vi "Dispose.vi"(8 "error in (no error)":errorcluster, 11 "TwinCAT ADS in":refnum<class "TwinCAT ADS.lvclass">) -> (0 "error out":errorcluster)   [LabVIEW 2018, in "TwinCAT ADS.lvclass"]
uses:
  TwinCAT ADS.lvclass
  TwinCAT ADS.lvclass/TwinCAT ADS.ctl
  TwinCAT.Ads
  Get Type Map.vi
  From Notification Key.vi
  Get Notification Map.vi
  Extensions/Delete Notification By Handle.vi
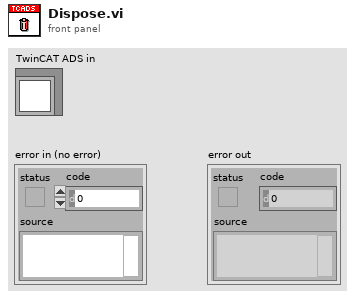
[diagram p1: front panel]
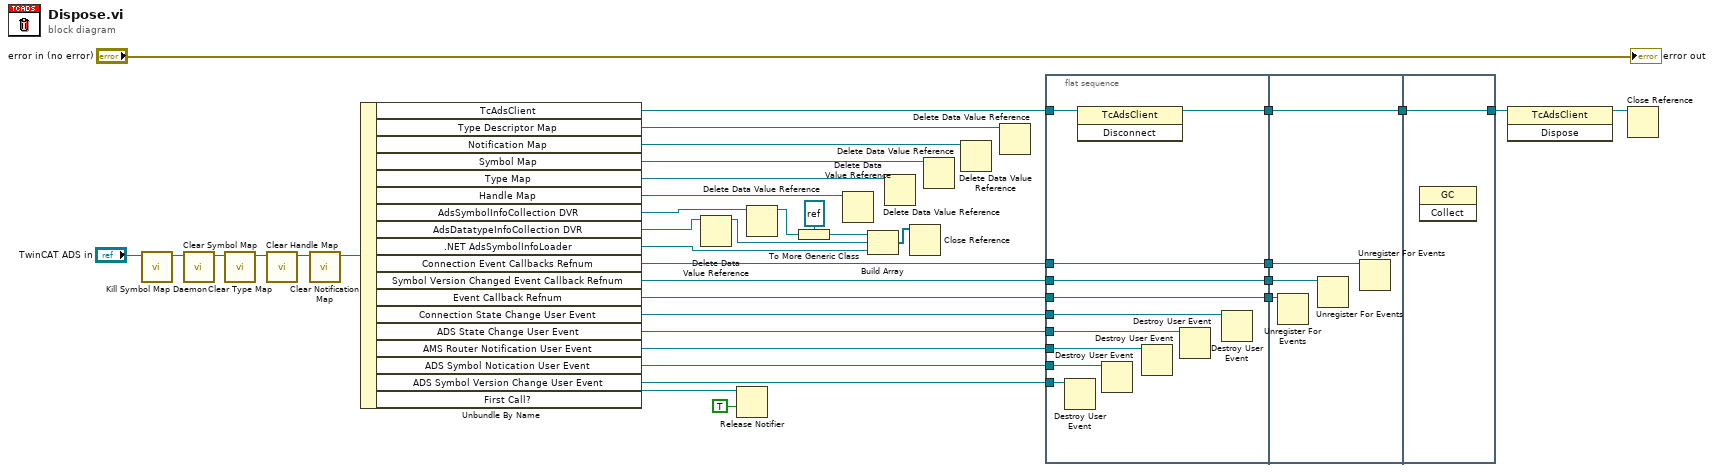
[diagram p0: block diagram]
diagram:
  n1 = call "Kill Symbol Map Daemon.vi"("TwinCAT ADS in"="TwinCAT ADS in") -> ("TwinCAT ADS out"=w3:refnum<class "TwinCAT ADS.lvclass">)  [unwired: 9 in, 1 out]
  n2 = call "Clear Symbol Map.vi"("TwinCAT ADS in"=w3) -> ("TwinCAT ADS out"=w35:refnum<class "TwinCAT ADS.lvclass">)  [unwired: 9 in, 1 out]
  n3 = call "Clear Type Map.vi"("TwinCAT ADS in"=w35) -> ("TwinCAT ADS out"=w34:refnum<class "TwinCAT ADS.lvclass">)  [unwired: 8 in, 2 out]
  n4 = call "Clear Handle Map.vi"("TwinCAT ADS in"=w34) -> ("TwinCAT ADS out"=w7:refnum<class "TwinCAT ADS.lvclass">)  [unwired: 9 in, 1 out]
  n5 = call "Clear Notification Map.vi"("TwinCAT ADS in"=w7) -> ("TwinCAT ADS out"=w6:refnum<class "TwinCAT ADS.lvclass">)  [unwired: 6 in, 4 out]
  n6 = Unbundle By Name(w6) -> ("TcAdsClient"=w26:refnum<k24>, "Type Descriptor Map"=w1:refnum<data-value>, "Notification Map"=w8:refnum<data-value>, "Symbol Map"=w9:refnum<data-value>, "Type Map"=w10:refnum<data-value>, "Handle Map"=w11:refnum<data-value>, "AdsSymbolInfoCollection DVR"=w12:refnum<data-value>, "AdsDatatypeInfoCollection DVR"=w13:refnum<data-value>, ".NET AdsSymbolInfoLoader"=w16:refnum<k24>, "Connection Event Callbacks Refnum"=w28:refnum<k27>, "Symbol Version Changed Event Callback Refnum"=w19:refnum<k27>, "Event Callback Refnum"=w29:refnum<k27>, "Connection State Change User Event"=w33:refnum<user-event>, "ADS State Change User Event"=w32:refnum<user-event>, "AMS Router Notification User Event"=w31:refnum<user-event>, "ADS Symbol Notication User Event"=w30:refnum<user-event>, "ADS Symbol Version Change User Event"=w17:refnum<user-event>, "First Call?"=w5:refnum<notifier>)
  n7 = Delete Data Value Reference(data value reference=w13) -> (data value=w14:refnum<k24>)  [unwired: 1 in, 1 out]
  n8 = Release Notifier(notifier=w5, force destroy? (F)=TRUE) -> ()  [unwired: 1 in, 3 out]
  n9 = Delete Data Value Reference(data value reference=w12) -> (data value=w15:refnum<k24>)  [unwired: 1 in, 1 out]
  n10 = To More Generic Class(target class=refnum<k24> refnum (".NET object"), reference=w15) -> (generic class reference=w37:refnum<k24>)
  n11 = Delete Data Value Reference(data value reference=w11) -> ()  [unwired: 1 in, 2 out]
  n12 = Build Array(w37, w14, w16) -> (w36:refnum<k24>[])
  n13 = Delete Data Value Reference(data value reference=w10) -> ()  [unwired: 1 in, 2 out]
  n14 = Close Reference(reference=w36) -> ()  [unwired: 1 in, 1 out]
  n15 = Delete Data Value Reference(data value reference=w9) -> ()  [unwired: 1 in, 2 out]
  n16 = Delete Data Value Reference(data value reference=w8) -> ()  [unwired: 1 in, 2 out]
  n17 = Delete Data Value Reference(data value reference=w1) -> ()  [unwired: 1 in, 2 out]
  n18 = flat-sequence {
    tunnel: w33 -> [w48]
    tunnel: w32 -> [w47]
    tunnel: w31 -> [w46]
    tunnel: w30 -> [w45]
    tunnel: w29 -> [w43]
    tunnel: w28 -> [w44]
    tunnel: w26 -> [w42]
    tunnel: [w44] -> w25
    tunnel: [w43] -> w24
    tunnel: [w41] -> w23
    tunnel: w19 -> [w40]
    tunnel: [w40] -> w18
    tunnel: w17 -> [w39]
    tunnel: w25 -> [w52]
    tunnel: w24 -> [w51]
    tunnel: w23 -> [w50]
    tunnel: [w50] -> w20
    tunnel: w18 -> [w49]
    tunnel: [w53] -> w21
    tunnel: w20 -> [w53]
    frame #0 {
      n19 = Destroy User Event(user event=w39) -> ()  [unwired: 1 in, 1 out]
      n20 = invoke class="TcAdsClient" method="Disconnect"(reference=w42) -> (reference out=w41:refnum<k24>)  [unwired: 2 in, 2 out]
      n21 = Destroy User Event(user event=w45) -> ()  [unwired: 1 in, 1 out]
      n22 = Destroy User Event(user event=w46) -> ()  [unwired: 1 in, 1 out]
      n23 = Destroy User Event(user event=w47) -> ()  [unwired: 1 in, 1 out]
      n24 = Destroy User Event(user event=w48) -> ()  [unwired: 1 in, 1 out]
    }
    frame #1 {
      n25 = Unregister For Events(event registration refnum=w51) -> ()  [unwired: 1 in, 1 out]
      n26 = Unregister For Events(event registration refnum=w49) -> ()  [unwired: 1 in, 1 out]
      n27 = Unregister For Events(event registration refnum=w52) -> ()  [unwired: 1 in, 1 out]
    }
    frame #2 {
      n28 = invoke class="GC" method="Collect"() -> ()  [unwired: 3 in, 3 out]
    }
  }
  n29 = invoke class="TcAdsClient" method="Dispose"(reference=w21) -> (reference out=w27:refnum<k24>)  [unwired: 2 in, 2 out]
  n30 = Close Reference(reference=w27) -> ()  [unwired: 1 in, 1 out]
  "error out" <- "error in (no error)"
